vi "calc_pol_scaling_params.vi"(0 "Min polarization":dbl, 11 "Max polarization":dbl) -> (4 "Minimum":dbl, 6 "Maximum":dbl, 8 "Increment":dbl, 10 "Minor increment":dbl, 15 "Start":dbl)   [LabVIEW 2015]
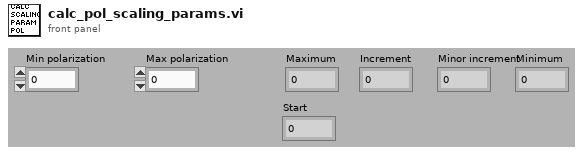
[diagram p1: front panel]
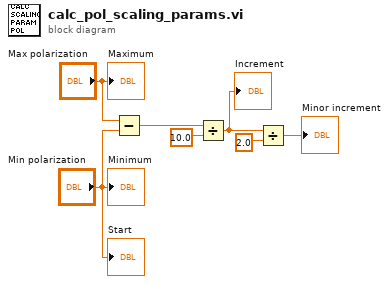
[diagram p0: block diagram]
diagram:
  n1 = Subtract(x="Max polarization", y="Min polarization") -> (x-y=w3:dbl)
  n2 = Divide(x=w3, y=10.0) -> (x/y=w5:dbl)
  "Increment" <- w5
  n3 = Divide(x=w5, y=2.0) -> (x/y=→"Minor increment":dbl)
  "Maximum" <- "Max polarization"
  "Minimum" <- "Min polarization"
  "Start" <- "Min polarization"
